vi "Demo_Graphiques.vi"() -> ()   [LabVIEW 2018]
panel:
  in  "Nb d'échantillons":i32=100
  out "XY Graph":cluster{u32[], dbl[]}(graph)
  out "Waveform Graph":dbl[](graph)
  out "Waveform Chart":dbl(graph)
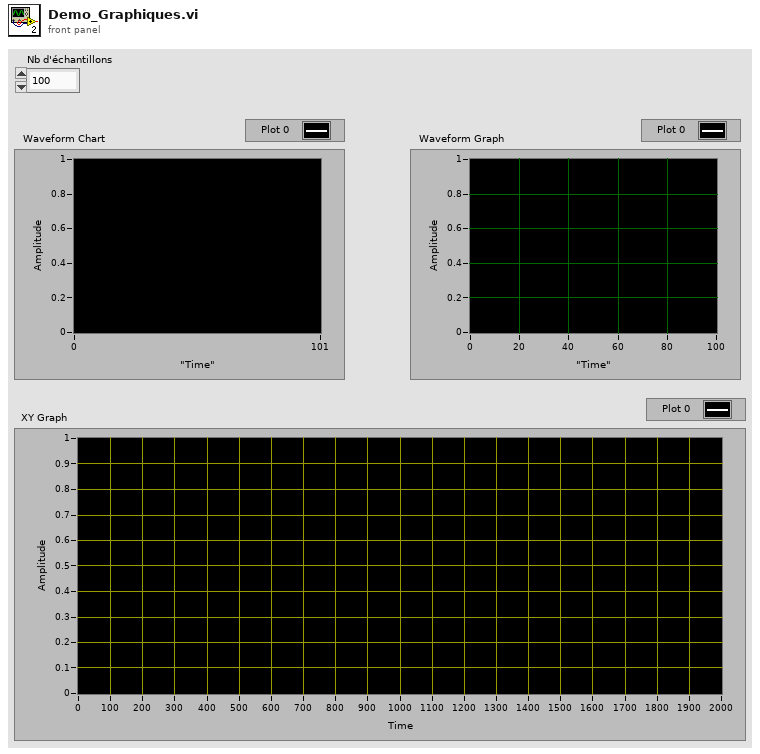
[diagram p1: front panel]
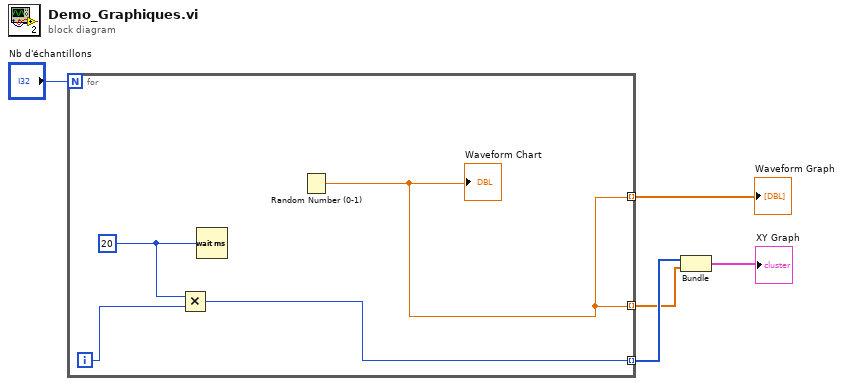
[diagram p0: block diagram]
diagram:
  n1 = for {
    N: "Nb d'échantillons" -> [_]
    tunnel: [w9] -> w5 mode=indexing
    tunnel: [w9] -> w1 mode=indexing
    tunnel: [w6] -> w2 mode=indexing
    i -> [w8]
    w7 = u32 20 ("milliseconds to wait")
    n2 = Multiply(x=w7, y=w8) -> (x*y=w6:u32)
    n3 = Wait (ms)(milliseconds to wait=w7) -> ()  [unwired: 1 out]
    n4 = Random Number (0-1)() -> (number: 0 to 1=w9:dbl)
    "Waveform Chart" <- w9
  }
  "Waveform Graph" <- w5
  n5 = Bundle(w2, w1) -> (→"XY Graph":cluster{u32[], dbl[]})  [unwired: 1 in]
